vi "Wrap Gyro Input.vi"(1 "In":dbl) -> (0 "Out":dbl)   [LabVIEW 2018]
doc: "Wraps gyro outputs and limits it to a -180 to 180 scale"
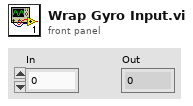
[diagram p1: front panel]
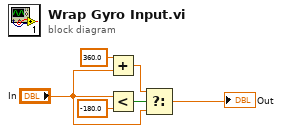
[diagram p0: block diagram]
diagram:
  n1 = Add(x=360.0, y="In") -> (x+y=w4:dbl)
  n2 = Less?(x="In", y=-180.0) -> (x < y?=w5:bool)
  n3 = Select(t=w4, s=w5, f="In") -> (s? t:f=→"Out":dbl)
